vi "GetHeatCameraInfo.vi"() -> ()   [LabVIEW 2020]
uses:
  <vilib>/httpClient/POSTBuffer.vi
  <vilib>/httpClient/LabVIEWHTTPClient.lvlib
panel:
  out "String":string
  out "Temperature (String)":string[](array[string])
  out "Temperatures":dbl[](array[numeric])
  in  "YPositions":dbl[](array[numeric])
  in  "XPositions":dbl[](array[numeric])
  out "Image":T1(plugin-control)
  in  "Array Type":dbl[](array[numeric])
  in  "Temperature Range (High)":dbl
  in  "Temperature Range (Low)":dbl
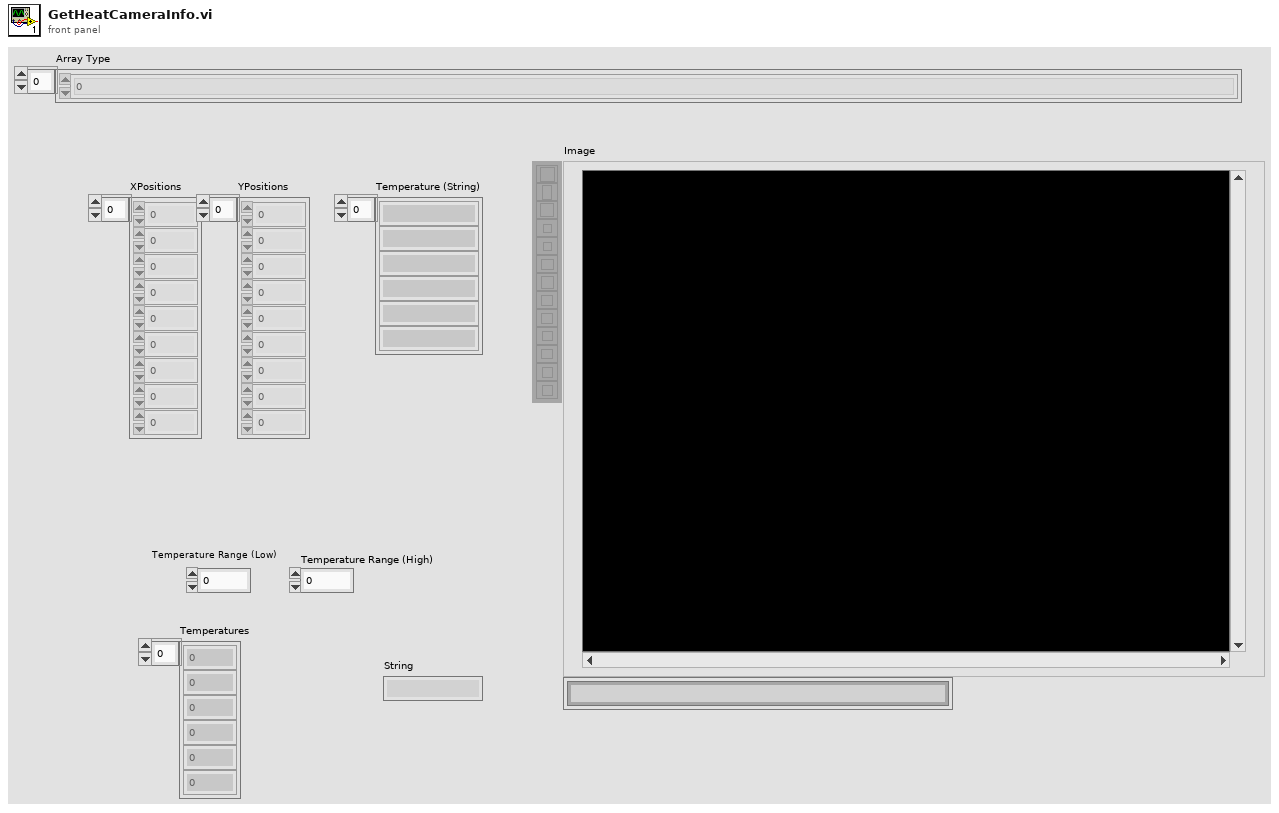
[diagram p1: front panel]
types:
  T1 = typedef "IMAQ Image.ctl" = refnum<image>
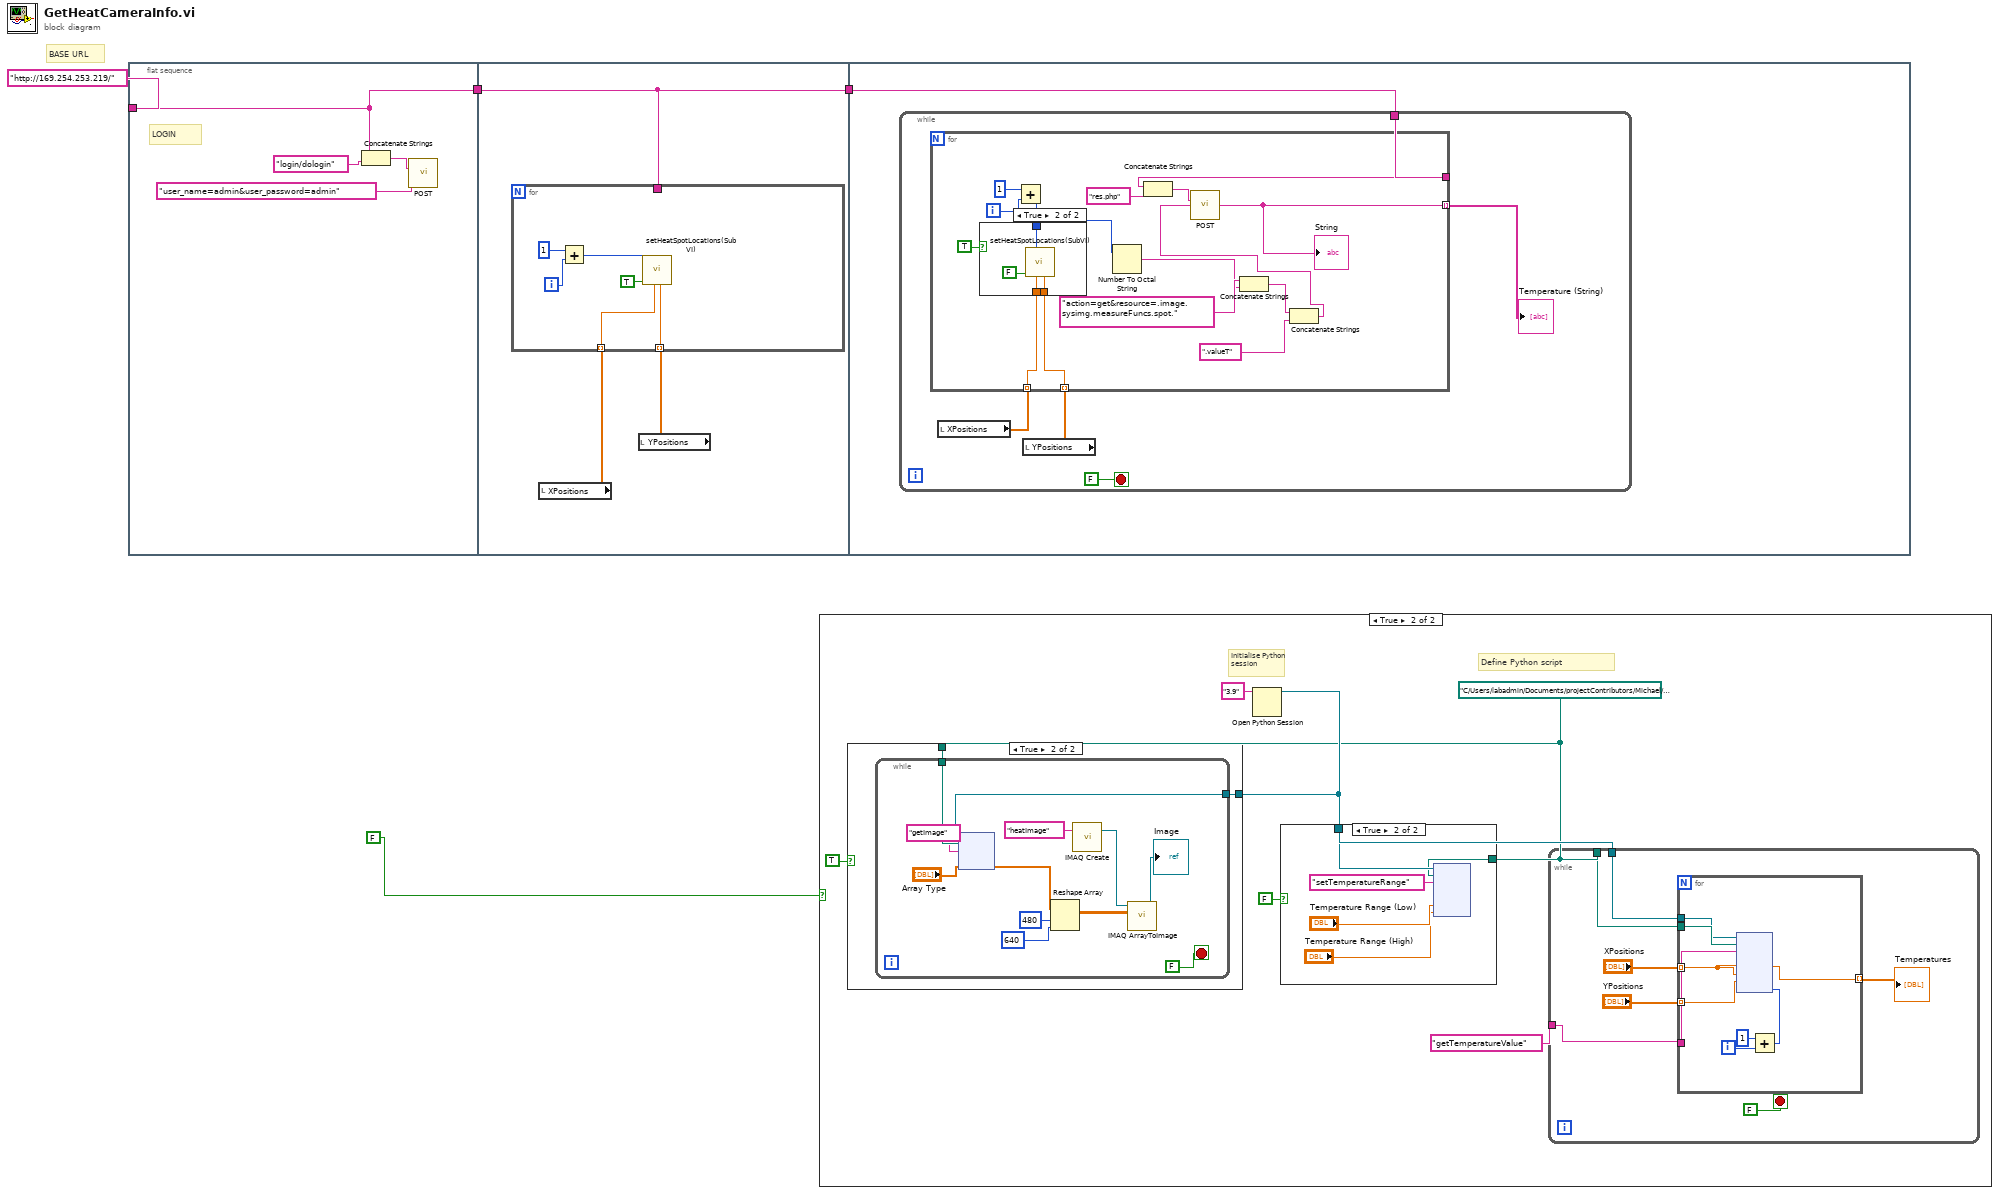
[diagram p0: block diagram]
diagram:
  # "BASE URL"
  n1 = flat-sequence {
    tunnel: "http://169.254.253.219/" ("url") -> [w5]
    tunnel: [w5] -> w2
    tunnel: w2 -> [w10]
    tunnel: [w10] -> w1
    tunnel: w1 -> [w18]
    frame #0 {
      # "LOGIN"
      n2 = Concatenate Strings(w5, "login/dologin" ("url")) -> (w6:string)
      n3 = call-poly <vilib>:"POST.vi"("url"=w6, "buffer"="user_name=admin&user_password=admin") -> ()  [unwired: 10 in, 4 out]
    }
    frame #1 {
      n4 = local read "XPositions"() -> (w11:dbl[])
      n5 = local read "YPositions"() -> (w9:dbl[])
      n6 = for {
        tunnel: w11 -> [w12] mode=indexing
        tunnel: w10 -> [_]
        tunnel: w9 -> [w13] mode=indexing
        i -> [w16]
        n7 = Add(x=1, y=w16) -> (x+y=w15:i32)
        n8 = call "setHeatSpotLocations(SubVI).vi"("YValue"=w13, "XValue"=w12, "Index"=w15, "Set active"=TRUE) -> ()  [unwired: 8 in]
      }
    }
    frame #2 {
      n9 = while {
        tunnel: w18 -> [w22]
        stop <- FALSE stop-if-true
        n10 = local read "XPositions"() -> (w19:dbl[])
        n11 = local read "YPositions"() -> (w20:dbl[])
        n12 = for {
          tunnel: w19 -> [w36] mode=indexing
          tunnel: w20 -> [w35] mode=indexing
          tunnel: w22 -> [w33]
          tunnel: [w27] -> w21 mode=indexing
          i -> [w38]
          n13 = Add(x=1, y=w38) -> (x+y=w31:i32)
          n14 = case shown="True" TRUE {
            tunnel: w36 -> [_ w42]
            tunnel: w35 -> [_ w41]
            tunnel: w31 -> [_ w40]
            frame False {
            }
            frame True {
              n15 = call "setHeatSpotLocations(SubVI).vi"("YValue"=w41, "XValue"=w42, "Index"=w40, "Set active"=FALSE) -> ()  [unwired: 8 in]
            }
          }
          n16 = Number To Octal String(2:w31) -> (0:w25:string)  [unwired: 1 in]
          n17 = Concatenate Strings(w33, "res.php" ("url")) -> (w34:string)
          n18 = Concatenate Strings("action=get&resource=.image.sysimg.measureFuncs.spot." ("buffer"), w25) -> (w30:string)
          n19 = Concatenate Strings(w30, ".valueT") -> (w28:string)
          n20 = call-poly <vilib>:"POST.vi"("url"=w34, "buffer"=w28) -> ("body"=w27:string)  [unwired: 10 in, 3 out]
          "String" <- w27
        }
        "Temperature (String)" <- w21
      }
    }
  }
  n21 = case shown="True" FALSE {
    frame False {
    }
    frame True {
      w45 = path "C:/Users/labadmin/Documents/projectContributors/Michael/multi-larva-cl-behavior-detection/LabViewSourceCode/heatCameraPythonCode/customFlir.py" ("module path")
      # "Define Python script"
      # "Initialise Python session"
      n22 = Open Python Session(python version="3.9" ("Python version")) -> (session out=w46:refnum<k35>)  [unwired: 2 in, 1 out]
      n23 = case shown="True" TRUE {
        tunnel: w46 -> [_ w55]
        tunnel: w45 -> [_ w54]
        frame False {
        }
        frame True {
          n24 = while {
            tunnel: w55 -> [w67]
            tunnel: w54 -> [w66]
            stop <- FALSE stop-if-true
            n25 = node(w67, w66, "getImage" ("function name"), "Array Type") -> (w63:dbl[])  [unwired: 1 in, 4 out]
            n26 = Reshape Array(w63, 480 ("dimension size"), 640 ("dimension size")) -> (w56:dbl[][])
            n27 = call "IMAQ Create"("Image Name"="heatImage") -> ("New Image"=w59:T1)  [unwired: 4 in, 1 out]
            n28 = call "IMAQ ArrayToImage"("Image Pixels (U8)"=w56, "Image"=w59) -> ("Image Out"=→"Image":T1)  [unwired: 8 in, 1 out]
          }
        }
      }
      n29 = case shown="True" FALSE {
        tunnel: w46 -> [_ w50]
        tunnel: w45 -> [_ w49]
        frame False {
        }
        frame True {
          n30 = node(w50, w49, "setTemperatureRange" ("function name"), "Temperature Range (Low)", "Temperature Range (High)") -> ()  [unwired: 5 in, 4 out]
        }
      }
      n31 = while {
        tunnel: w45 -> [w74]
        tunnel: w46 -> [w73]
        tunnel: "getTemperatureValue" ("function name") -> [w72]
        stop <- FALSE stop-if-true
        n32 = for {
          tunnel: w74 -> [w83]
          tunnel: w73 -> [w82]
          tunnel: w72 -> [w81]
          tunnel: "XPositions" -> [w80] mode=indexing
          tunnel: "YPositions" -> [w79] mode=indexing
          tunnel: [w75] -> w68 mode=indexing
          i -> [w78]
          n33 = Add(x=1, y=w78) -> (x+y=w76:i32)
          n34 = node(w82, w83, w81, w80, w80, w79, w76) -> (w75:dbl)  [unwired: 4 in, 4 out]
        }
        "Temperatures" <- w68
      }
    }
  }
